vi "Com_Matrix220_Initialize.vi"(8 "error in":errorcluster, 10 "Remote Port":u16=51236, 11 "IP Address":string="192.168.3.100") -> (0 "error out":errorcluster, 3 "Buffer Data":T1)   [LabVIEW 2016]
uses:
  Data Def/Com_Matrix220_Buffer Data.ctl
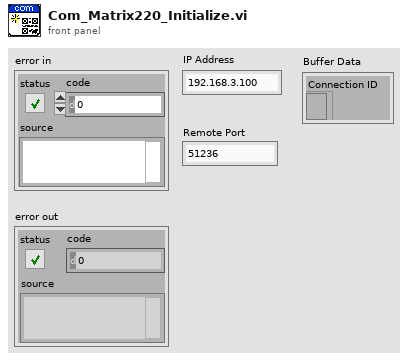
[diagram p1: front panel]
types:
  T1 = typedef "Com_Matrix220_Buffer Data.ctl" = cluster{"Connection ID":refnum<k5>}
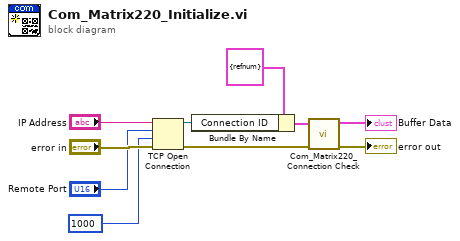
[diagram p0: block diagram]
diagram:
  n1 = TCP Open Connection(address="IP Address", remote port or service name="Remote Port", timeout ms (60000)=1000, error in (no error)="error in") -> (connection ID=w5:refnum<k5>, error out=w4:errorcluster)  [unwired: 1 in]
  n2 = Bundle By Name(cluster=T1 {"Connection ID"=refnum} ("Buffer Data"), "Connection ID"=w5) -> (w3:T1)
  n3 = call "Com_Matrix220_Connection Check.vi"("error in"=w4, "Buffer Data In"=w3) -> ("error out"=→"error out":errorcluster, "Buffer Data Out"=→"Buffer Data":T1)  [unwired: 7 in, 1 out]
